vi "Calculate Protection Value.vi"(5 "Payload Length":u32, 7 "Frame ID":u32, 8 "error in (no error)":errorcluster, 9 "Overrides":dbl[](array[numeric]), 10 "Frame.Data in":dbl[](array[numeric]), 11 "Protection Configuration in":T1 {"CRC Channels"."Data Type" items=["Signed", "Unsigned", "IEEE Float"]}) -> (0 "error out":errorcluster, 1 "Protection Value":dbl, 2 "Frame.Data out":dbl[](array[numeric]), 3 "Protection Configuration out":T1 {"CRC Channels"."Data Type" items=["Signed", "Unsigned", "IEEE Float"]})   [LabVIEW 2019, in "Protection and Counter Support Engine.lvlib"]
uses:
  Protection and Counter Support Engine.lvlib
  Types/RT Protection Configuration.ctl
  Shared/Types/Protection Type.ctl
  Shared/Types/XNET Signal Configuration.ctl
  <vilib>/xnet/xnet.llb/XNET Convert (Signal to Frame Raw).vi
  Shared/Protection and Counter Support Shared.lvlib
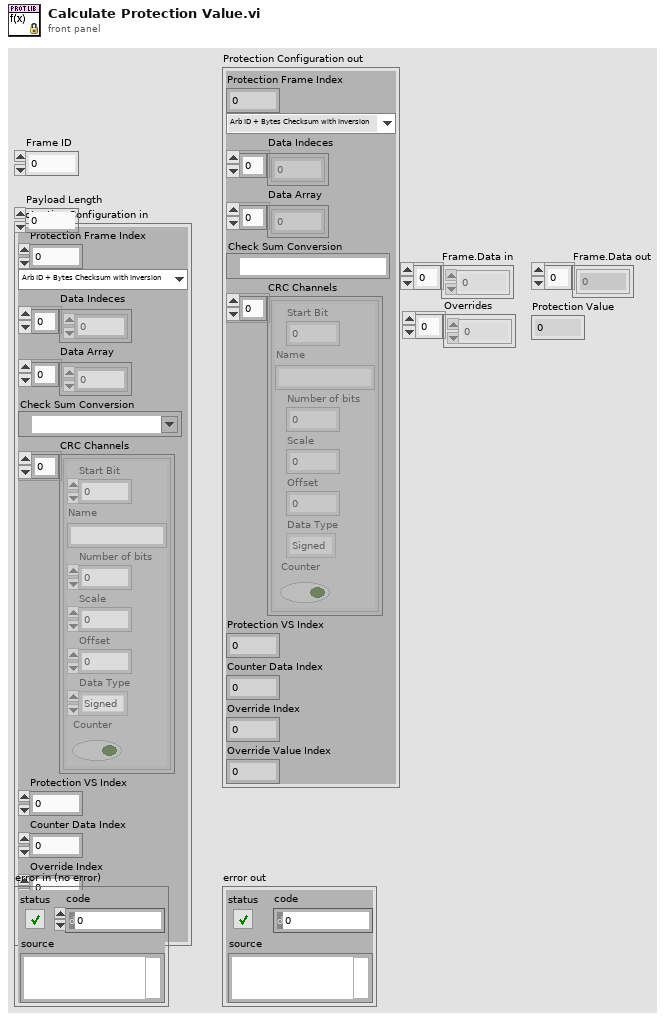
[diagram p1: front panel]
types:
  T1 = typedef "Protection and Counter Support Engine.lvlib/RT Protection Configuration.ctl" = cluster{"Protection Frame Index":i32, "Protection Type":T2, "Data Indeces":i32[], "Data Array":dbl[], "Check Sum Conversion":refnum<k21>, "CRC Channels":T3[], "Protection VS Index":i32, "Counter Data Index":i32, "Override Index":i32, "Override Value Index":i32}
  T2 = typedef "Protection and Counter Support Shared.lvlib/Protection Type.ctl" = enum16{"Arb ID + Bytes Checksum with Inversion", "Arb ID + Bytes CRC with Inversion", "Reversed Raw Signal Checksum with Inversion", "Concatenated Two's Compliment"}
  T3 = typedef "Protection and Counter Support Shared.lvlib/XNET Signal Configuration.ctl" = cluster{"Start Bit":i32, "Name":string, "Number of bits":i32, "Scale":dbl, "Offset":dbl, "Data Type":u32, "Counter":bool}
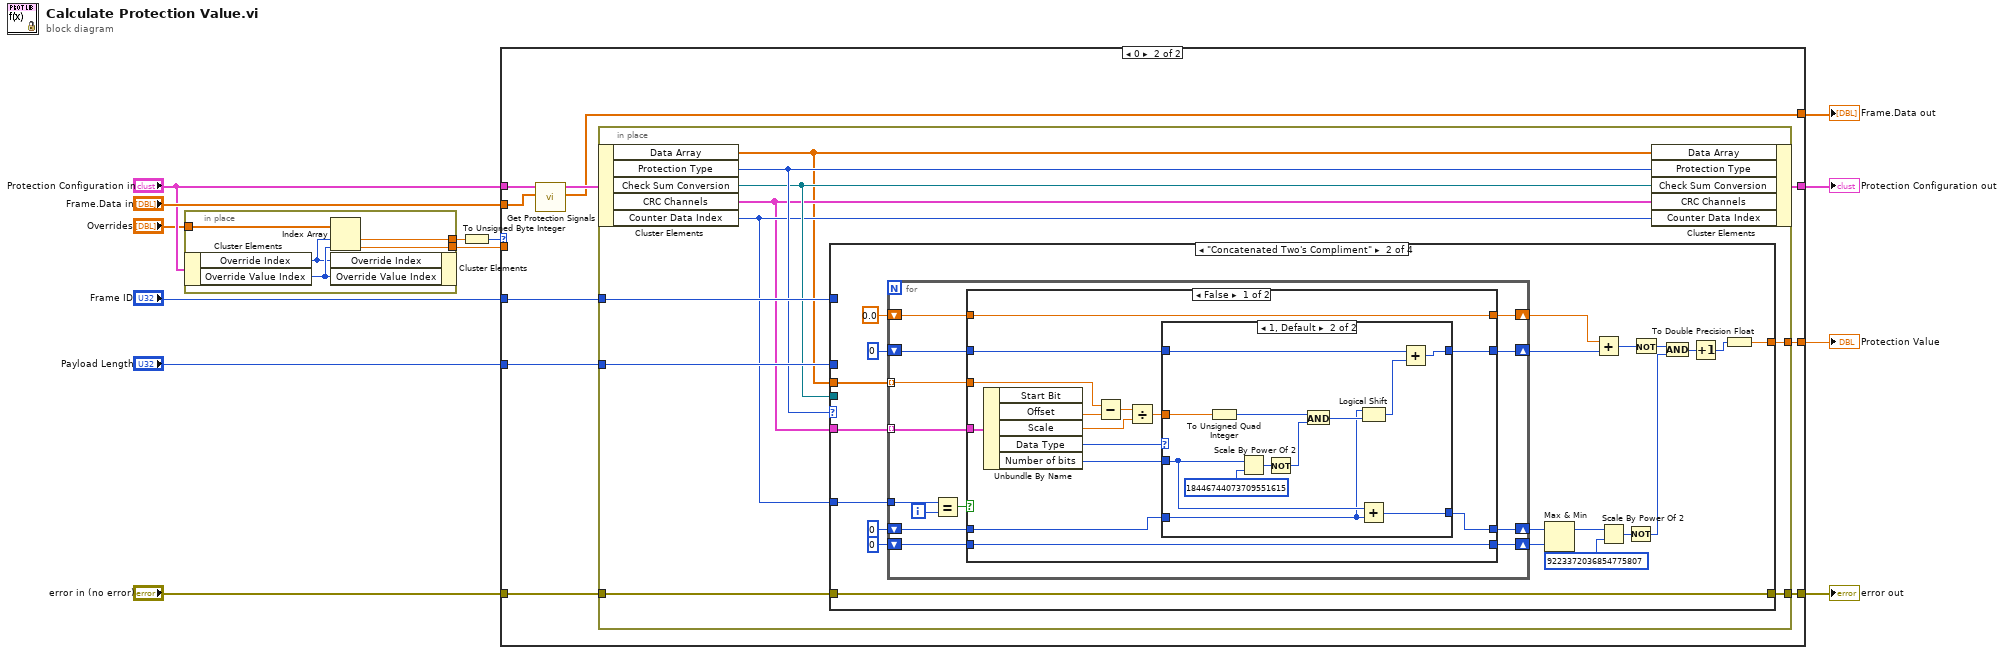
[diagram p0: block diagram]
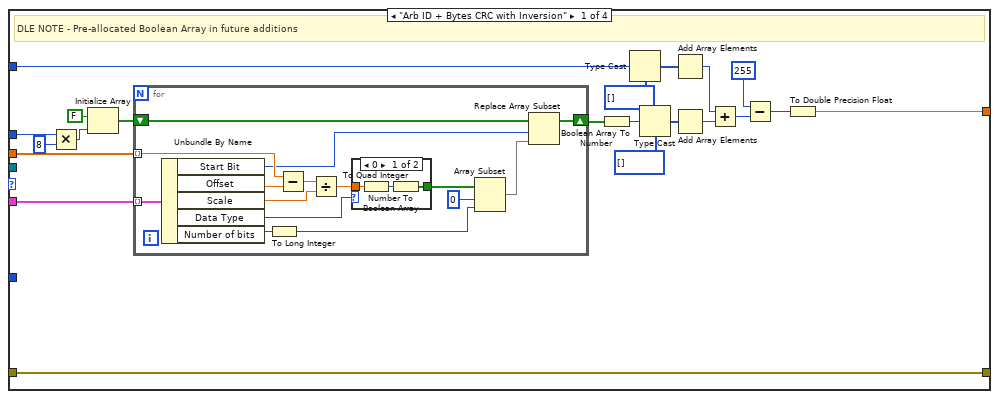
[diagram p3: hidden frame]
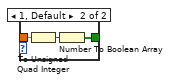
[diagram p4: hidden frame]
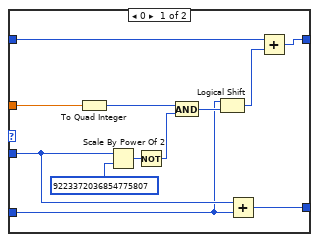
[diagram p5: hidden frame]
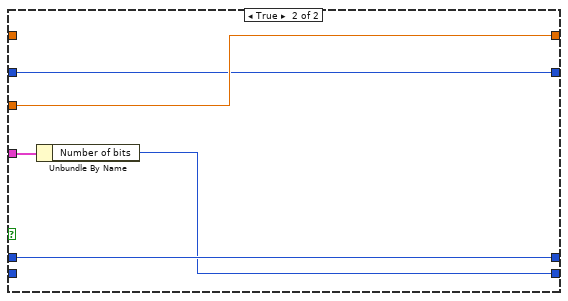
[diagram p6: hidden frame]
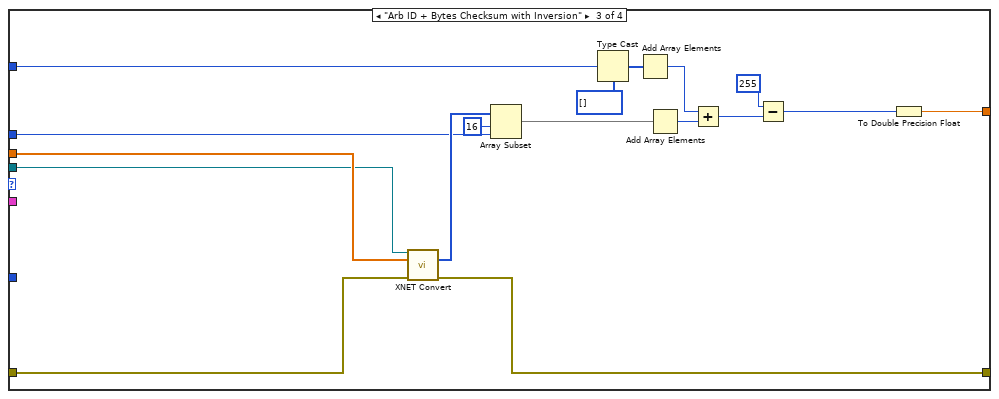
[diagram p7: hidden frame]
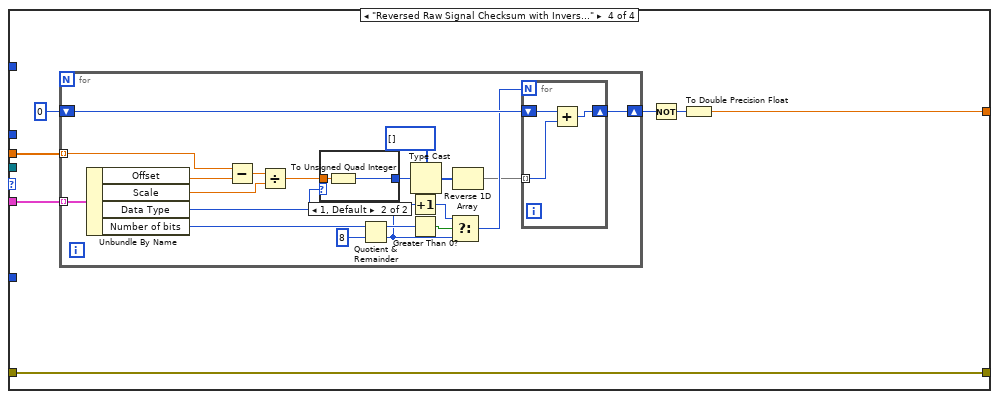
[diagram p8: hidden frame]
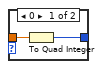
[diagram p9: hidden frame]
diagram:
  n1 = in-place {
    in-place-border: "Overrides" -> [w18]
    in-place-border: [w15] -> w3
    in-place-border: [w14] -> w1
    n2 = in-place-cluster #1("Protection Configuration in") -> ("Override Index"=w16:i32, "Override Value Index"=w17:i32)
    n3 = Index Array(array=w18, index #1=w16, index #2=w17) -> (element #1=w15:dbl, element #2=w14:dbl)
    n4 = in-place-cluster #1("Override Index"=w16, "Override Value Index"=w17) -> ()  [unwired: 1 out]
  }
  n5 = To Unsigned Byte Integer(number=w3) -> (unsigned 8bit integer=w2:u8)
  n6 = case shown="0" w2 {
    tunnel: "Payload Length" -> [_ w32]
    tunnel: "error in (no error)" -> [w19 w31]
    tunnel: "Frame ID" -> [_ w30]
    tunnel: [w22 w28] -> w10
    tunnel: "Frame.Data in" -> [w20 w27]
    tunnel: [w21 w26] -> w8
    tunnel: [w20 w25] -> w7
    tunnel: [w19 w24] -> w6
    tunnel: "Protection Configuration in" -> [w21 w23]
    tunnel: w1 -> [w22 _]
    frame Default {
    }
    frame 0 {
      n7 = call "Get Protection Signals.vi"("Frame.Data in"=w27, "Protection Configuration"=w23) -> ("Frame.Data out"=w25:dbl[], "Protection Configuration out"=w29:T1)  [unwired: 8 in]
      n8 = in-place {
        in-place-border: w30 -> [w42]
        in-place-border: w31 -> [w41]
        in-place-border: w32 -> [w40]
        in-place-border: [w39] -> w24
        in-place-border: [w38] -> w28
        n9 = in-place-cluster #2(w29) -> ("Data Array"=w33:dbl[], "Protection Type"=w37:T2, "Check Sum Conversion"=w36:refnum<k21>, "CRC Channels"=w34:T3[], "Counter Data Index"=w35:i32)
        n10 = case shown="\"Concatenated Two's Compliment\"" w37 {
          tunnel: w42 -> [w61 _ w176 _]
          tunnel: [w43 w104 w162 w179] -> w38
          tunnel: w41 -> [w52 w105 w170 w180]
          tunnel: [w52 w105 w169 w180] -> w39
          tunnel: w34 -> [w50 w87 _ w183]
          tunnel: w33 -> [w51 w86 w166 w182]
          tunnel: w36 -> [_ _ w165 _]
          tunnel: w40 -> [w46 _ w163 _]
          tunnel: w35 -> [_ w92 _ _]
          frame "Arb ID + Bytes CRC with Inversion" {
            # "DLE NOTE - Pre-allocated Boolean Array in future additions"
            n11 = Multiply(x=w46, y=u32 8) -> (x*y=w45:u32)
            n12 = Initialize Array(FALSE, w45) -> (w49:bool[])
            n13 = for {
              tunnel: w50 -> [w78] mode=indexing
              shift-right: [w69] -> w55
              shift-left: w49 -> [w71]
              tunnel: w51 -> [w68] mode=indexing
              n14 = Unbundle By Name(w78) -> ("Start Bit"=w65:i32, "Offset"=w77:dbl, "Scale"=w75:dbl, "Data Type"=w67:u32, "Number of bits"=w73:i32)
              n15 = To Long Integer(number=w73) -> (32bit integer=w64:i32)
              n16 = Subtract(x=w68, y=w77) -> (x-y=w76:dbl)
              n17 = Divide(x=w76, y=w75) -> (x/y=w74:dbl)
              n18 = case shown="0" w67 {
                tunnel: w74 -> [w81 w84]
                tunnel: [w79 w82] -> w66
                frame 0 {
                  n19 = To Quad Integer(1:w81) -> (0:w80:i64)
                  n20 = Number To Boolean Array(number=w80) -> (Boolean array=w79:bool[])
                }
                frame 1, Default {
                  n21 = To Unsigned Quad Integer(1:w84) -> (0:w83:u64)
                  n22 = Number To Boolean Array(number=w83) -> (Boolean array=w82:bool[])
                }
              }
              n23 = Array Subset(array=w66, index=0, length=w64) -> (w70:bool[])
              n24 = Replace Array Subset(array=w71, new element=w70, index=w65) -> (w69:bool[])
            }
            n25 = Boolean Array To Number(Boolean array=w55) -> (number=w54:u64)
            n26 = Type Cast(type=u8[] [], x=w61) -> (*(type *) &x=w60:u8[])
            n27 = Type Cast(type=u8[] [], x=w54) -> (*(type *) &x=w47:u8[])
            n28 = Add Array Elements(numeric array=w60) -> (sum=w59:u8)
            n29 = Add Array Elements(numeric array=w47) -> (sum=w63:u8)
            n30 = Add(x=w59, y=w63) -> (x+y=w58:u8)
            n31 = Subtract(x=u8 255, y=w58) -> (x-y=w56:u8)
            n32 = To Double Precision Float(number=w56) -> (double precision float=w43:dbl)
          }
          frame "Concatenated Two's Compliment" {
            n33 = for {
              tunnel: w87 -> [w118] mode=indexing
              shift-right: [w113] -> w101
              shift-left: i64 0 -> [w116]
              tunnel: w86 -> [w117] mode=indexing
              shift-right: [w115] -> w96
              shift-left: i64 0 -> [w114]
              tunnel: w92 -> [w112]
              shift-right: [w107] -> w89
              shift-left: 0.0 -> [w109]
              shift-right: [w106] -> w88
              shift-left: i64 0 -> [w108]
              i -> [w111]
              n34 = Equal?(x=w112, y=w111) -> (x = y?=w110:bool)
              n35 = case shown="False" w110 {
                tunnel: w118 -> [w132 w161]
                tunnel: w117 -> [w127 w160]
                tunnel: w116 -> [w124 w159]
                tunnel: [w123 w158] -> w115
                tunnel: w114 -> [w122 w158]
                tunnel: [w121 w159] -> w113
                tunnel: w109 -> [w119 _]
                tunnel: w108 -> [w120 _]
                tunnel: [w119 w160] -> w107
                tunnel: [w120 w157] -> w106
                frame False {
                  n36 = Unbundle By Name(w132) -> ("Offset"=w131:dbl, "Scale"=w129:dbl, "Data Type"=w126:u32, "Number of bits"=w125:i32)  [unwired: 1 out]
                  n37 = Subtract(x=w127, y=w131) -> (x-y=w130:dbl)
                  n38 = Divide(x=w130, y=w129) -> (x/y=w128:dbl)
                  n39 = case shown="1, Default" w126 {
                    tunnel: w128 -> [w144 w154]
                    tunnel: w125 -> [w137 w150]
                    tunnel: w124 -> [w139 w148]
                    tunnel: [w136 w149] -> w123
                    tunnel: w122 -> [w134 w145]
                    tunnel: [w135 w146] -> w121
                    frame 0 {
                      n40 = To Quad Integer(1:w144) -> (0:w141:i64)
                      n41 = Scale By Power Of 2(n=w137, x=i64 9223372036854775807 ("n")) -> (x*2^n=w143:i64)
                      n42 = Not(x=w143) -> (.not. x?=w140:i64)
                      n43 = And(x=w141, y=w140) -> (x .and. y?=w138:i64)
                      n44 = Logical Shift(y=w134, x=w138) -> (x << y=w133:i64)
                      n45 = Add(x=w137, y=w134) -> (x+y=w136:i64)
                      n46 = Add(x=w139, y=w133) -> (x+y=w135:i64)
                    }
                    frame 1, Default {
                      n47 = To Unsigned Quad Integer(1:w154) -> (0:w153:u64)
                      n48 = Scale By Power Of 2(n=w150, x=u64 18446744073709551615 ("n")) -> (x*2^n=w156:u64)
                      n49 = Not(x=w156) -> (.not. x?=w152:u64)
                      n50 = And(x=w153, y=w152) -> (x .and. y?=w151:u64)
                      n51 = Logical Shift(y=w145, x=w151) -> (x << y=w147:u64)
                      n52 = Add(x=w150, y=w145) -> (x+y=w149:i64)
                      n53 = Add(x=w148, y=w147) -> (x+y=w146:i64)
                    }
                  }
                }
                frame True {
                  n54 = Unbundle By Name(w161) -> ("Number of bits"=w157:i32)
                }
              }
            }
            n55 = Max & Min(x=w96, y=w88) -> (max(x,y)=w85:i64)  [unwired: 1 out]
            n56 = Add(x=w89, y=w101) -> (x+y=w100:i64)
            n57 = Scale By Power Of 2(n=w85, x=i64 9223372036854775807 ("n")) -> (x*2^n=w98:i64)
            n58 = Not(x=w98) -> (.not. x?=w97:i64)
            n59 = Not(x=w100) -> (.not. x?=w95:i64)
            n60 = And(x=w95, y=w97) -> (x .and. y?=w94:i64)
            n61 = Increment(x=w94) -> (x+1=w99:i64)
            n62 = To Double Precision Float(number=w99) -> (double precision float=w104:dbl)
          }
          frame "Arb ID + Bytes Checksum with Inversion" {
            n63 = call-poly <vilib>:"XNET Convert.vi"("session in"=w165, "signal data"=w166, "error in (no error)"=w170) -> ("frame data"=w167:u8[], "error out"=w169:errorcluster)  [unwired: 10 in, 1 out]
            n64 = Array Subset(array=w167, index=16 ("length"), length=w163) -> (w164:u8[])
            n65 = Type Cast(type=u8[] [], x=w176) -> (*(type *) &x=w175:u8[])
            n66 = Add Array Elements(numeric array=w175) -> (sum=w174:u8)
            n67 = Add Array Elements(numeric array=w164) -> (sum=w178:u8)
            n68 = Add(x=w174, y=w178) -> (x+y=w173:u8)
            n69 = Subtract(x=u8 255, y=w173) -> (x-y=w171:u8)
            n70 = To Double Precision Float(number=w171) -> (double precision float=w162:dbl)
          }
          frame "Reversed Raw Signal Checksum with Inversion" {
            n71 = for {
              tunnel: w183 -> [w205] mode=indexing
              tunnel: w182 -> [w202] mode=indexing
              shift-right: [w199] -> w184
              shift-left: u8 0 -> [w200]
              n72 = Unbundle By Name(w205) -> ("Offset"=w204:dbl, "Scale"=w203:dbl, "Data Type"=w201:u32, "Number of bits"=w197:i32)
              n73 = Subtract(x=w202, y=w204) -> (x-y=w196:dbl)
              n74 = Divide(x=w196, y=w203) -> (x/y=w195:dbl)
              n75 = case shown="1, Default" w201 {
                tunnel: w195 -> [w210 w212]
                tunnel: [w209 w211] -> w198
                frame 0 {
                  n76 = To Quad Integer(1:w210) -> (0:w209:i64)
                }
                frame 1, Default {
                  n77 = To Unsigned Quad Integer(1:w212) -> (0:w211:u64)
                }
              }
              n78 = Quotient & Remainder(x=w197, y=8) -> (x-y*floor(x/y)=w192:i32, floor(x/y)=w190:i32)
              n79 = Increment(x=w190) -> (x+1=w191:i32)
              n80 = Greater Than 0?(x=w192) -> (x > 0?=w193:bool)
              n81 = Type Cast(type=u8[] [], x=w198) -> (*(type *) &x=w187:u8[])
              n82 = Select(t=w191, s=w193, f=w190) -> (s? t:f=w189:i32)
              n83 = Reverse 1D Array(array=w187) -> (reversed array=w186:u8[])
              n84 = for {
                N: w189 -> [_]
                tunnel: w186 -> [w207] mode=indexing
                shift-right: [w206] -> w199
                shift-left: w200 -> [w208]
                n85 = Add(x=w208, y=w207) -> (x+y=w206:u8)
              }
            }
            n86 = Not(x=w184) -> (.not. x?=w181:u8)
            n87 = To Double Precision Float(number=w181) -> (double precision float=w179:dbl)
          }
        }
        n88 = in-place-cluster #2("Data Array"=w33, "Protection Type"=w37, "Check Sum Conversion"=w36, "CRC Channels"=w34, "Counter Data Index"=w35) -> (w26:T1)
      }
    }
  }
  "Protection Configuration out" <- w8
  "error out" <- w6
  "Frame.Data out" <- w7
  "Protection Value" <- w10
